vi "sub_hw-err-checking.vi"(7 "cmd":enum16{"write", "read", "init"}(ring), 11 "check hw status in":T1) -> (3 "check hw status out":T1)   [LabVIEW 2019]
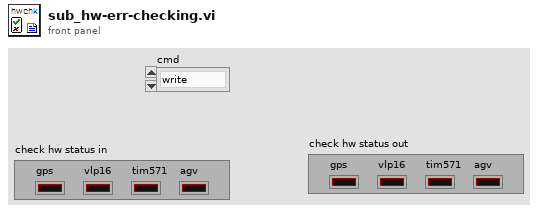
[diagram p1: front panel]
types:
  T1 = cluster{"gps":bool, "vlp16":bool, "tim571":bool, "agv":bool}
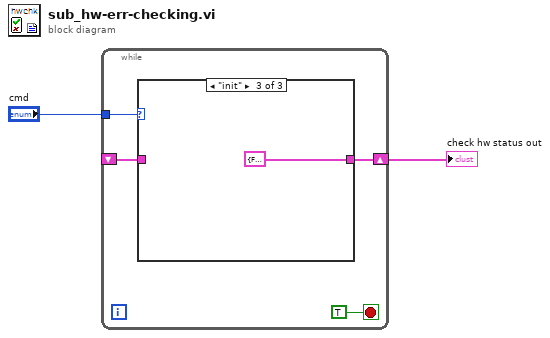
[diagram p0: block diagram]
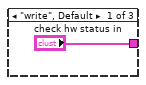
[diagram p2: hidden frame]
diagram:
  n1 = while {
    tunnel: "cmd" -> [w5]
    shift-right: [w4] -> w1
    shift-left: _ -> [w3]
    stop <- TRUE stop-if-true
    n2 = case shown="\"init\"" w5 {
      tunnel: ["check hw status in" w8 T1 {"gps"=FALSE, "vlp16"=FALSE, "tim571"=FALSE, "agv"=FALSE} ("check hw status in")] -> w4
      tunnel: w3 -> [_ w8 _]
      frame "write", Default {
      }
      frame "read" {
      }
      frame "init" {
      }
    }
  }
  "check hw status out" <- w1
